vi "Entradas Analogicas.vi"() -> ()   [LabVIEW 2023]
uses:
  <vilib>/Instr/_visa.llb/VISA Configure Serial Port (Instr).vi
panel:
  out "Waveform Chart 2":dbl(graph)
  out "Tank 2":dbl(slide) scale=0.0..3.3
  out "Gauge 2":dbl(knob) scale=0.0..10.0
  out "Valor analogico 2":dbl
  out "Meter 2":ext(knob) scale=0.0..3.3
  out "Waveform Chart":dbl(graph)
  out "Tank":dbl(slide) scale=0.0..3.3
  out "Gauge":dbl(knob) scale=0.0..10.0
  out "Valor analogico":dbl
  in  "stop":bool
  in  "VISA resource name":refnum<visa-resource-name>
  out "Meter":ext(knob) scale=0.0..3.3
  # "Medidor de voltaje"
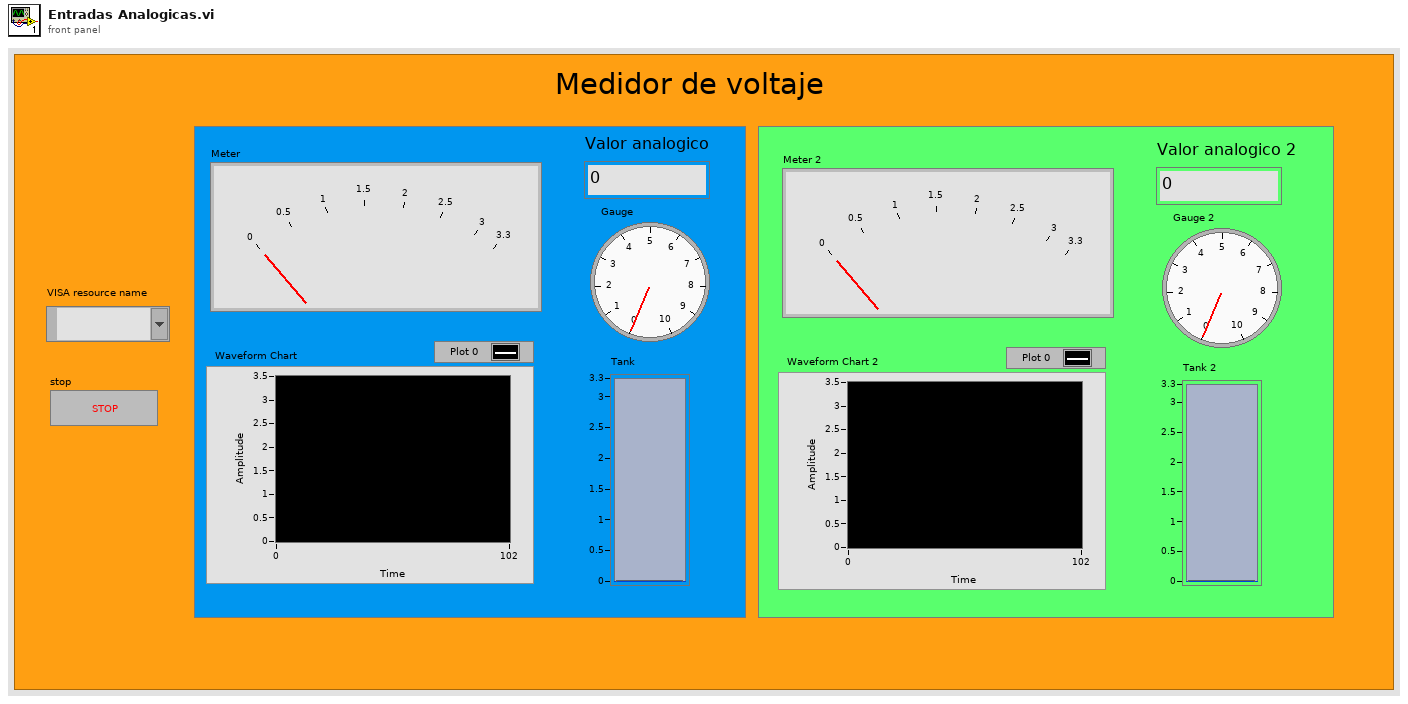
[diagram p1: front panel]
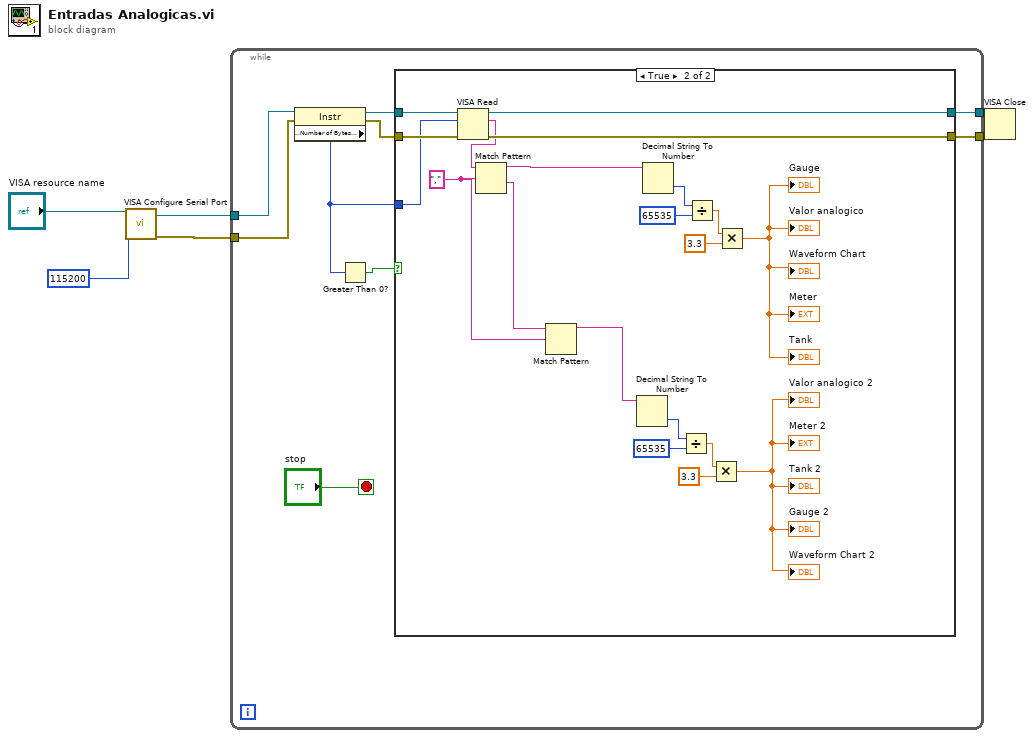
[diagram p0: block diagram]
diagram:
  n1 = call-poly "VISA Configure Serial Port"("VISA resource name"="VISA resource name", "baud rate (9600)"=u32 115200) -> ("VISA resource name out"=w4:refnum<visa-resource-name>, "error out"=w3:errorcluster)  [unwired: 12 in]
  n2 = while {
    tunnel: w4 -> [w14]
    tunnel: w3 -> [w13]
    tunnel: [w10] -> w2
    tunnel: [w9] -> w1
    stop <- "stop" stop-if-true
    n3 = property class="Instr"(reference=w14, error in=w13) -> (reference out=w12:refnum<visa-resource-name>, error out=w11:errorcluster, "Serial Settings:Number of Bytes at Serial Port"=w7:u32)
    n4 = Greater Than 0?(x=w7) -> (x > 0?=w8:bool)
    n5 = case shown="True" w8 {
      tunnel: w12 -> [w17 w37]
      tunnel: w11 -> [w16 w36]
      tunnel: [w17 w35] -> w10
      tunnel: [w16 w34] -> w9
      tunnel: w7 -> [_ w18]
      frame False {
      }
      frame True {
        w19 = "," ("regular expression")
        n6 = VISA Read(VISA resource name=w37, byte count=w18, error in (no error)=w36) -> (VISA resource name out=w35:refnum<visa-resource-name>, read buffer=w33:string, error out=w34:errorcluster)  [unwired: 1 out]
        n7 = Match Pattern(string=w33, regular expression=w19) -> (before substring=w22:string, after substring=w23:string)  [unwired: 1 in, 2 out]
        n8 = Match Pattern(string=w23, regular expression=w19) -> (before substring=w24:string)  [unwired: 1 in, 3 out]
        n9 = Decimal String To Number(string=w24) -> (number=w25:i32)  [unwired: 2 in, 1 out]
        n10 = Decimal String To Number(string=w22) -> (number=w29:i32)  [unwired: 2 in, 1 out]
        n11 = Divide(x=w25, y=65535) -> (x/y=w27:dbl)
        n12 = Divide(x=w29, y=65535) -> (x/y=w31:dbl)
        n13 = Multiply(x=w27, y=3.3) -> (x*y=→"Meter 2" →"Valor analogico 2" →"Gauge 2" →"Tank 2" →"Waveform Chart 2":dbl)
        n14 = Multiply(x=w31, y=3.3) -> (x*y=→"Gauge" →"Valor analogico" →"Waveform Chart" →"Meter" →"Tank":dbl)
      }
    }
  }
  n15 = VISA Close(VISA resource name=w2, error in (no error)=w1) -> ()  [unwired: 1 out]
